vi "Configure Bus Definition (Bits Mask).vi"(8 "error in (no error)":errorcluster, 9 "Mask (FFFF)":i32=65535 format="%x", 10 "Bus Name (1: Digital Bus 1)":i32(ring)=1 items=["Digital Bus 1"=1, "Digital Bus 2"=2], 11 "VISA resource name":refnum<visa-resource-name>) -> (0 "error out":errorcluster, 3 "VISA resource name out":refnum<visa-resource-name>)   [LabVIEW 2015, in "Agilent 2000 3000 X-Series.lvlib"]
doc: "Configures the digital bus definition in bit mask mode."
uses:
  <instrlib>/Agilent 2000 3000 X-Series/Agilent 2000 3000 X-Series.lvlib
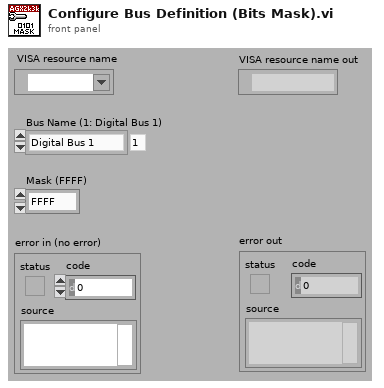
[diagram p1: front panel]
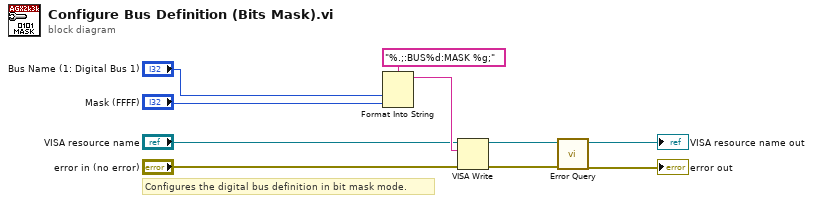
[diagram p0: block diagram]
diagram:
  # "Configures the digital bus definition in bit mask mode."
  n1 = Format Into String(format string="%.;:BUS%d:MASK %g;", "Bus Name (1: Digital Bus 1)", "Mask (FFFF)") -> (resulting string=w8:string)  [unwired: 2 in, 1 out]
  n2 = VISA Write(VISA resource name="VISA resource name", write buffer=w8, error in (no error)="error in (no error)") -> (VISA resource name out=w5:refnum<visa-resource-name>, error out=w4:errorcluster)  [unwired: 1 out]
  n3 = call <instrlib>:"Error Query.vi"("error in (no error)"=w4, "VISA resource name"=w5) -> ("error out"=→"error out":errorcluster, "VISA resource name out"=→"VISA resource name out":refnum<visa-resource-name>)  [unwired: 8 out]
